vi "Kafka_ConsumerExitLoop.vi"(8 "error in (no error)":errorcluster, 11 "Consumer Handle":string="localhost:9092") -> (0 "error out":errorcluster, 3 "Consumer Handle":string)   [LabVIEW 2019]
uses:
  VS2017/KafkaLVLib/x64/Debug/KafkaLVLib.dll
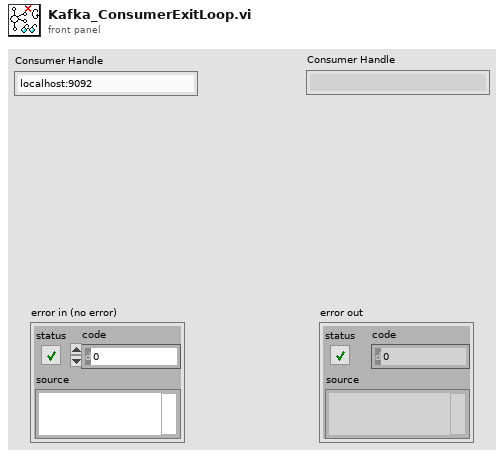
[diagram p1: front panel]
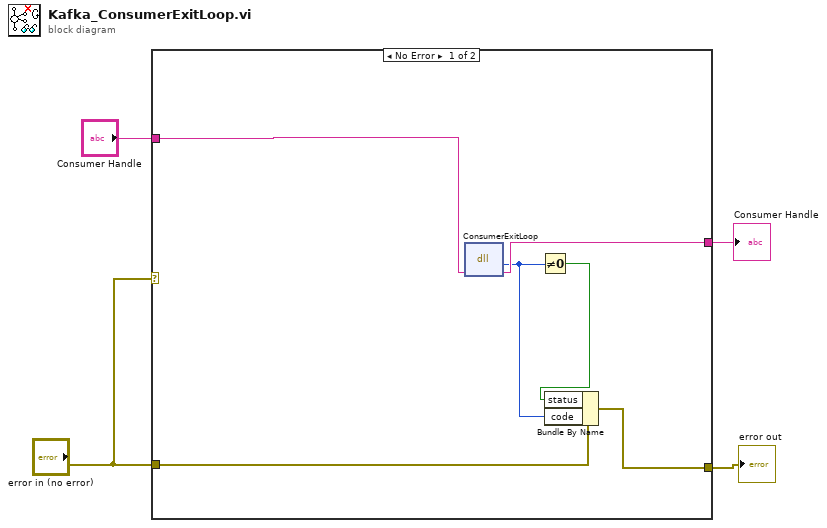
[diagram p0: block diagram]
diagram:
  n1 = case shown="No Error" "error in (no error)" {
    tunnel: "error in (no error)" -> [w10 w12]
    tunnel: "Consumer Handle" -> [w9 w11]
    tunnel: [w8 w12] -> w3
    tunnel: [w7 w11] -> w2
    frame No Error {
      n2 = dll-call lib="C:/Users/schandho/OneDrive - National Instruments/Research/Virtualization/SemiADV/KafkaLVLib/VS2017/KafkaLVLib/x64/Debug/KafkaLVLib.dll" fn="ConsumerExitLoop"("consumerhandle"=w9) -> ("error"=w5:i32, "consumerhandle"=w7:string)  [unwired: 3 in, 2 out]
      n3 = Not Equal To 0?(x=w5) -> (x != 0?=w6:bool)
      n4 = Bundle By Name(cluster=w10, "status"=w6, "code"=w5) -> (w8:errorcluster)
    }
    frame Error {
    }
  }
  "error out" <- w3
  "Consumer Handle" <- w2
